vi "OutBitsCheckCommands.vi"(0 "outBit0":bool, 2 "outBit1":bool, 4 "outBit2":bool, 6 "actStep":i32, 8 "stepChanged":bool, 10 "actScan":i32, 12 "scanChanged":bool) -> (14 "outBit0out":bool, 16 "outBit1out":bool, 18 "outBit2out":bool)   [LabVIEW 2014]
uses:
  OutbitsGlobalVars.vi
  <vilib>/rvi/Emulation/niFpgaGetClockAttributes.vi
  <vilib>/rvi/Emulation/niFpgaSctlEmulationGetInTimedLoop.vi
  <vilib>/rvi/Emulation/niFpgaEmulationReportErrorSimple.vi
  <vilib>/rvi/Memory/Memory_Emulation/nirvimemoryFastEmulation.vi
  <vilib>/rvi/Memory/Memory_Emulation/nirvimemoryEmulation.vi
  <vilib>/rvi/Emulation/niFpgaEmulationIsFPGAContextNoSignature.vi
  <vilib>/rvi/DataTransferAndStorage/Container/Common/niFpgaContainerGetUniqueNameForEmu.vi
  <vilib>/rvi/Emulation/niFpgaProcessEmulError.vi
  <vilib>/rvi/errors/nirviReportUnexpectedCaseInternalError (U32).vi
  <vilib>/rvi/Emulation/niFpgaCriticalErrorInLSC.vi
  <vilib>/rvi/DataTransferAndStorage/Container/XNode/niFpgaContainer.xnode
panel:
  # "This will loop over all cmds in memory and check\nif for this step or scan any command for this outbit is set\n and will change the output accordingly"
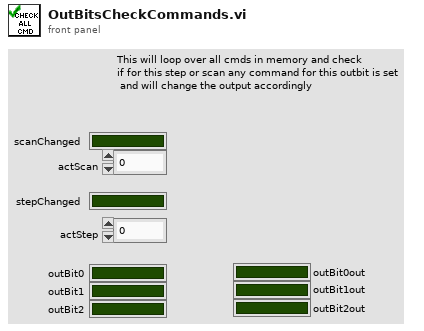
[diagram p1: front panel]
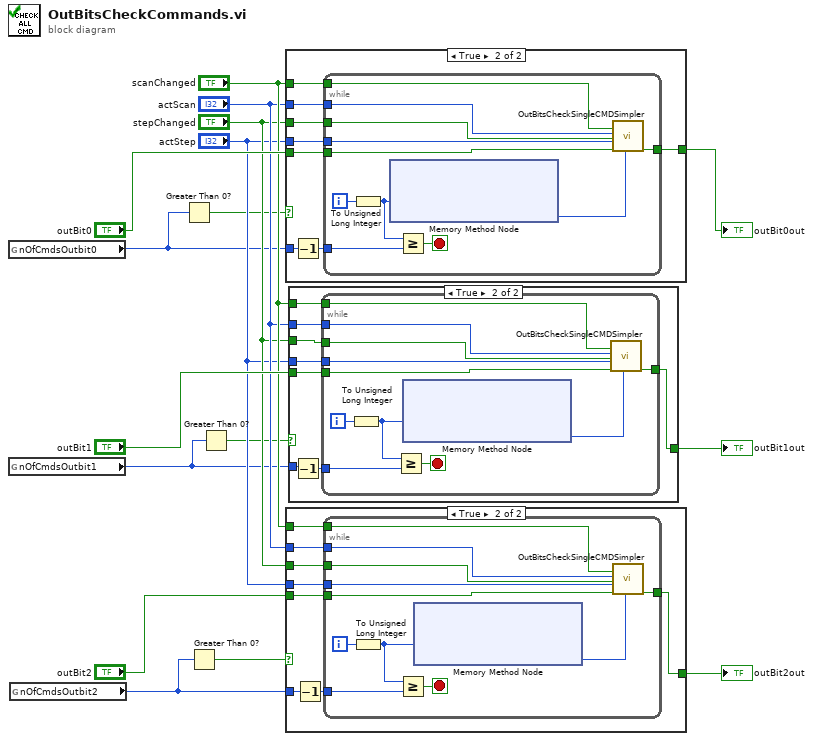
[diagram p0: block diagram]
diagram:
  n1 = global read "OutbitsGlobalVars.vi" "nOfCmdsOutbit0"() -> (w6:u32)
  n2 = global read "OutbitsGlobalVars.vi" "nOfCmdsOutbit1"() -> (w4:u32)
  n3 = global read "OutbitsGlobalVars.vi" "nOfCmdsOutbit2"() -> (w2:u32)
  n4 = Greater Than 0?(x=w6) -> (x > 0?=w5:bool)
  n5 = Greater Than 0?(x=w2) -> (x > 0?=w1:bool)
  n6 = Greater Than 0?(x=w4) -> (x > 0?=w3:bool)
  n7 = case shown="True" w5 {
    tunnel: w6 -> [_ w25]
    tunnel: "outBit0" -> [w17 w23]
    tunnel: [w17 w22] -> w15
    tunnel: "scanChanged" -> [_ w21]
    tunnel: "actScan" -> [_ w20]
    tunnel: "stepChanged" -> [_ w19]
    tunnel: "actStep" -> [_ w18]
    frame False {
    }
    frame True {
      n8 = Decrement(x=w25) -> (x-1=w24:u32)
      n9 = while {
        tunnel: w24 -> [w34]
        tunnel: w21 -> [w31]
        tunnel: w20 -> [w30]
        tunnel: w19 -> [w29]
        tunnel: w18 -> [w28]
        tunnel: w23 -> [w27]
        tunnel: [w26] -> w22
        i -> [w36]
        stop <- w33 stop-if-true
        n10 = To Unsigned Long Integer(number=w36) -> (unsigned 32bit integer=w35:u32)
        n11 = xnode ("Memory Method Node")("Address"=w35) -> ("Data"=w32:u32)  [unwired: 1 in, 1 out]
        n12 = Greater Or Equal?(x=w35, y=w34) -> (x >= y?=w33:bool)
        n13 = call "OutBitsCheckSingleCMDSimpler.vi"("scanChanged"=w31, "actScan"=w30, "stepChanged"=w29, "actStep"=w28, "outbit_in"=w27, "CMDin"=w32) -> ("outbit_out"=w26:bool)  [unwired: 13 in]
      }
    }
  }
  "outBit0out" <- w15
  n14 = case shown="True" w1 {
    tunnel: "scanChanged" -> [_ w45]
    tunnel: "actScan" -> [_ w44]
    tunnel: "stepChanged" -> [_ w43]
    tunnel: "actStep" -> [_ w42]
    tunnel: w2 -> [_ w41]
    tunnel: "outBit2" -> [w37 w39]
    tunnel: [w37 w38] -> w7
    frame False {
    }
    frame True {
      n15 = Decrement(x=w41) -> (x-1=w40:u32)
      n16 = while {
        tunnel: w40 -> [w55]
        tunnel: w45 -> [w53]
        tunnel: w44 -> [w52]
        tunnel: w43 -> [w51]
        tunnel: w42 -> [w50]
        tunnel: w39 -> [w49]
        tunnel: [w48] -> w38
        i -> [w56]
        stop <- w54 stop-if-true
        n17 = To Unsigned Long Integer(number=w56) -> (unsigned 32bit integer=w47:u32)
        n18 = Greater Or Equal?(x=w47, y=w55) -> (x >= y?=w54:bool)
        n19 = xnode ("Memory Method Node")("Address"=w47) -> ("Data"=w46:u32)  [unwired: 1 in, 1 out]
        n20 = call "OutBitsCheckSingleCMDSimpler.vi"("scanChanged"=w53, "actScan"=w52, "stepChanged"=w51, "actStep"=w50, "outbit_in"=w49, "CMDin"=w46) -> ("outbit_out"=w48:bool)  [unwired: 13 in]
      }
    }
  }
  "outBit2out" <- w7
  n21 = case shown="True" w3 {
    tunnel: "outBit1" -> [w57 w65]
    tunnel: w4 -> [_ w64]
    tunnel: "scanChanged" -> [_ w62]
    tunnel: "actScan" -> [_ w61]
    tunnel: "stepChanged" -> [_ w60]
    tunnel: "actStep" -> [_ w59]
    tunnel: [w57 w58] -> w8
    frame False {
    }
    frame True {
      n22 = Decrement(x=w64) -> (x-1=w63:u32)
      n23 = while {
        tunnel: w63 -> [w75]
        tunnel: w62 -> [w73]
        tunnel: w61 -> [w72]
        tunnel: w60 -> [w71]
        tunnel: w59 -> [w70]
        tunnel: w65 -> [w69]
        tunnel: [w68] -> w58
        i -> [w76]
        stop <- w74 stop-if-true
        n24 = To Unsigned Long Integer(number=w76) -> (unsigned 32bit integer=w67:u32)
        n25 = Greater Or Equal?(x=w67, y=w75) -> (x >= y?=w74:bool)
        n26 = xnode ("Memory Method Node")("Address"=w67) -> ("Data"=w66:u32)  [unwired: 1 in, 1 out]
        n27 = call "OutBitsCheckSingleCMDSimpler.vi"("scanChanged"=w73, "actScan"=w72, "stepChanged"=w71, "actStep"=w70, "outbit_in"=w69, "CMDin"=w66) -> ("outbit_out"=w68:bool)  [unwired: 13 in]
      }
    }
  }
  "outBit1out" <- w8
